vi "Setup.vi"(11 "Sound Demo.lvclass":refnum<class "Sound Demo.lvclass">) -> (0 "error out":errorcluster, 3 "Sound Demo.lvclass out":refnum<class "Sound Demo.lvclass">)   [LabVIEW 2010, in "Sound Demo.lvclass"]
doc: "Select which sound player should be used for the demo."
uses:
  Sound Demo.lvclass
  Select Sound Player.ctl
  Sound Player/Sound Player.lvclass
  Sound Demo.lvclass/Sound Demo.ctl
panel:
  in  "Select sound player:":T1 items=["Sound Card", "Sound Visualizer"]
  in  "Cancel":bool
  in  "OK":bool
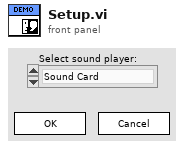
[diagram p1: front panel]
types:
  T1 = typedef "Sound Demo.lvclass/Select Sound Player.ctl" = u16
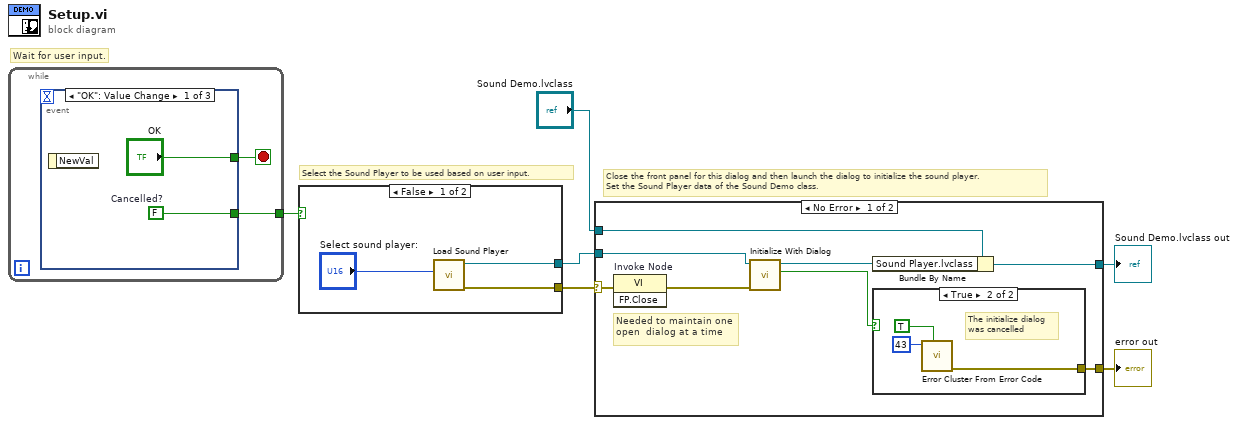
[diagram p0: block diagram]
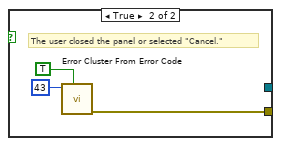
[diagram p4: hidden frame]
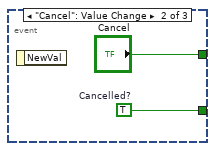
[diagram p5: hidden frame]
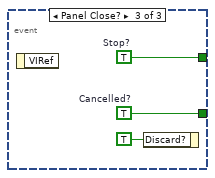
[diagram p6: hidden frame]
diagram:
  # "Close the front panel for this dialog and then launch the dialog to initialize the sound player.\nSet the Sound Player data of the Sound Demo class."
  # "Select the Sound Player to be used based on user input."
  # "Wait for user input."
  n1 = while {
    tunnel: [w7] -> w6
    stop <- w8 stop-if-true
    n2 = event shown="[0] \"OK\": Value Change" {
      selector: _ -> [_ _ _]
      dyn-events: _ -> [_ _ _]
      timeout: _ -> [_ _ _]
      tunnel: ["OK" "Cancel" w14] -> w8
      tunnel: [w10 w12 w13] -> w7
      event "OK": Value Change {
        w10 = FALSE  # Cancelled?
        n3 = event-data() -> ()  [unwired: 1 in, 1 out]
      }
      event "Cancel": Value Change {
        w12 = TRUE  # Cancelled?
        n4 = event-data() -> ()  [unwired: 1 in, 1 out]
      }
      event Panel Close? {
        w13 = TRUE  # Cancelled?
        w14 = TRUE  # Stop?
        n5 = event-data() -> ()  [unwired: 1 in, 1 out]
        n6 = event-data("Discard?"=TRUE) -> ()  [unwired: 1 in, 1 out]
      }
    }
  }
  n7 = case shown="False" w6 {
    tunnel: [w16 w19] -> w5
    tunnel: [w17 _] -> w4
    frame False {
      n8 = call "Load Sound Player.vi"("Select sound player:"="Select sound player:") -> ("error out"=w16:errorcluster, "Sound Player out"=w17:refnum<class "Sound Player.lvclass">)  [unwired: 9 in]
    }
    frame True {
      # "The user closed the panel or selected \"Cancel.\""
      n9 = call <vilib>:"Error Cluster From Error Code.vi"("show call chain? (False)"=TRUE, "error code (0)"=43) -> ("error out"=w19:errorcluster)  [unwired: 7 in]
    }
  }
  n10 = case shown="No Error" w5 {
    selector: w5 -> [w23 w33]
    tunnel: w4 -> [w29 _]
    tunnel: "Sound Demo.lvclass" -> [w27 w34]
    tunnel: [w26 w34] -> w2
    tunnel: [w24 w33] -> w1
    frame No Error {
      # "Needed to maintain one open  dialog at a time"
      n11 = invoke on="Invoke Node" class="VI" method="FP.Close"(error in=w23) -> (error out=w22:errorcluster)  [unwired: 2 in, 2 out]
      n12 = call-dynamic "Initialize With Dialog.vi"("error in (no error)"=w22, "Sound Player in"=w29) -> ("Cancelled?"=w25:bool, "Sound Player out"=w28:refnum<class "Sound Player.lvclass">)  [unwired: 7 in, 1 out]
      n13 = Bundle By Name "Bundle By Name"(cluster=w27, "Sound Player.lvclass"=w28) -> (w26:refnum<class "Sound Demo.lvclass">)
      n14 = case shown="True" w25 {
        tunnel: [_ w30] -> w24
        frame False {
          # "The initialize dialog was NOT cancelled."
        }
        frame True {
          # "The initialize dialog\nwas cancelled"
          n15 = call <vilib>:"Error Cluster From Error Code.vi"("show call chain? (False)"=TRUE, "error code (0)"=43) -> ("error out"=w30:errorcluster)  [unwired: 7 in]
        }
      }
    }
    frame Error {
    }
  }
  "Sound Demo.lvclass out" <- w2
  "error out" <- w1
